vi "TRABS-calc-2017-SD-correc.vi"(3 "II channel seq":T1, 4 "minmaxOD":cluster{"ODmin":dbl, "ODmax":dbl}, 5 "I channel seq":T1) -> (0 "Finished":bool=TRUE, 1 "diffpoints":i32, 2 "TRABS":dbl[][](array[numeric]))   [LabVIEW 2015]
uses:
  controls/data-cluster.ctl
  globalVarSD.vi
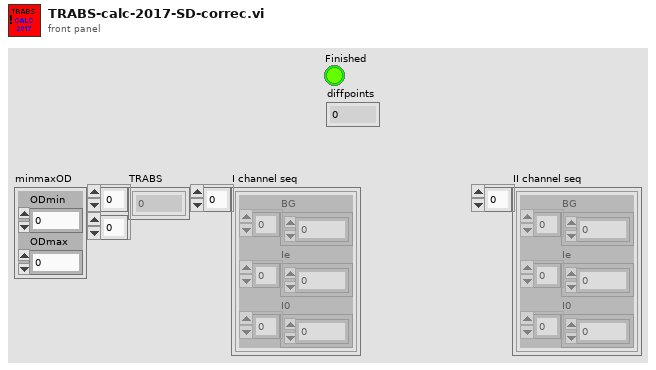
[diagram p1: front panel]
types:
  T1 = typedef "data-cluster.ctl" = cluster{"BG":i32[], "Ie":i32[], "I0":i32[]}[]
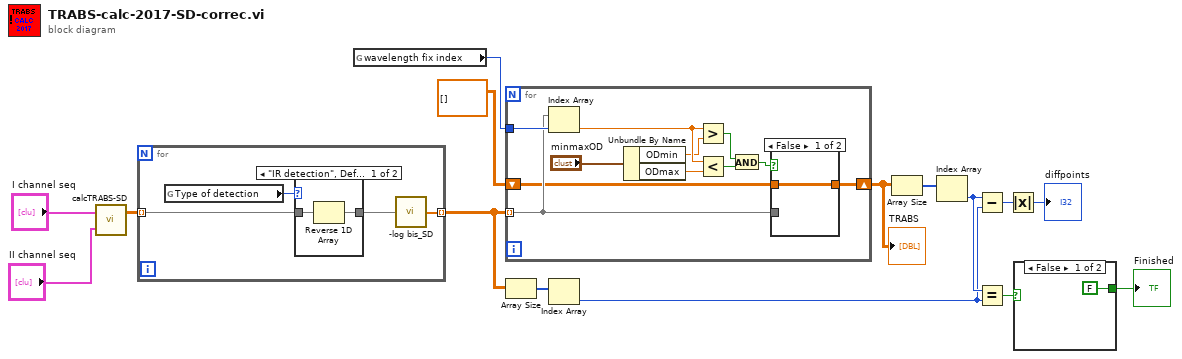
[diagram p0: block diagram]
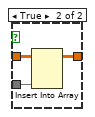
[diagram p2: hidden frame]
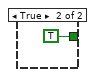
[diagram p3: hidden frame]
diagram:
  n1 = call "calcTRABS-SD.vi"("II channel seq"="II channel seq", "I channel seq"="I channel seq") -> ("TRanS multiple measurements"=w2:dbl[][])  [unwired: 1 out]
  n2 = for {
    tunnel: w2 -> [w17] mode=indexing
    tunnel: [w19] -> w10 mode=indexing
    n3 = global read "globalVarSD.vi" "Type of detection"() -> (w18:enum32{"IR detection", "UV-vis detection"})
    n4 = case shown="\"IR detection\", Default" w18 {
      tunnel: w17 -> [w21 w22]
      tunnel: [w20 w22] -> w16
      frame "IR detection", Default {
        n5 = Reverse 1D Array(array=w21) -> (reversed array=w20:dbl[])
      }
      frame "UV-vis detection" {
      }
    }
    n6 = call "-log bis_SD.vi"("Transmission"=w16) -> ("-log(x)=log(1/x)"=w19:dbl[])
  }
  n7 = global read "globalVarSD.vi" "wavelength fix index"() -> (w12:i16)
  n8 = for {
    tunnel: w10 -> [w27] mode=indexing
    tunnel: w12 -> [w29]
    shift-right: [w25] -> w1
    shift-left: dbl[][] [] ("-log(x)=log(1/x)") -> [w26]
    n9 = Index Array(array=w27, index=w29) -> (element=w31:dbl)
    n10 = Unbundle By Name("minmaxOD") -> ("ODmin"=w24:dbl, "ODmax"=w23:dbl)
    n11 = Greater?(x=w31, y=w24) -> (0:w33:bool)
    n12 = Less?(x=w31, y=w23) -> (x < y?=w32:bool)
    n13 = And(x=w33, y=w32) -> (x .and. y?=w28:bool)
    n14 = case shown="False" w28 {
      tunnel: w27 -> [_ w36]
      tunnel: w26 -> [w34 w37]
      tunnel: [w34 w35] -> w25
      frame False {
      }
      frame True {
        n15 = Insert Into Array(array=w37, new element=w36) -> (w35:dbl[][])  [unwired: 2 in]
      }
    }
  }
  "TRABS" <- w1
  n16 = Array Size(array=w10) -> (size(s)=w8:i32[])
  n17 = Index Array(array=w8) -> (element=w5:i32)  [unwired: 1 in]
  n18 = Array Size(array=w1) -> (size(s)=w9:i32[])
  n19 = Index Array(array=w9) -> (element=w6:i32)  [unwired: 1 in]
  n20 = Subtract(x=w6, y=w5) -> (x-y=w4:i32)
  n21 = Equal?(x=w6, y=w5) -> (x = y?=w7:bool)
  n22 = Absolute Value(x=w4) -> (abs(x)=→"diffpoints":i32)
  n23 = case shown="False" w7 {
    tunnel: [FALSE TRUE] -> w13
    frame False {
    }
    frame True {
    }
  }
  "Finished" <- w13
